vi "GetShortcuts.vi"(8 "error in (no error)":errorcluster, 11 "menu in":refnum<class "menu.lvclass">) -> (0 "error out":errorcluster, 2 "shortcuts":string[](array[string]), 3 "menu out":refnum<class "menu.lvclass">)   [LabVIEW 2009, in "menu.lvclass"]
uses:
  menu.lvclass
  menu.lvclass/menu.ctl
  Menu Item/menu item.lvclass
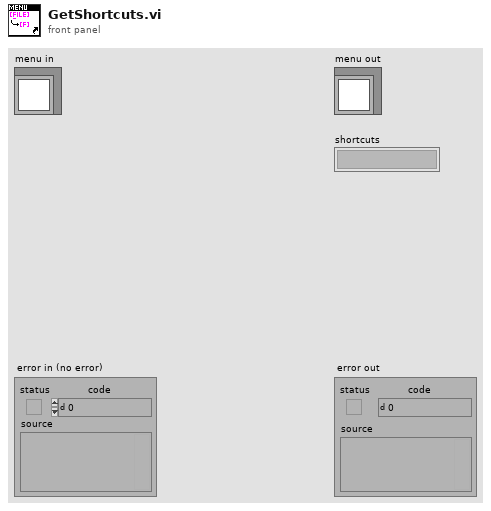
[diagram p1: front panel]
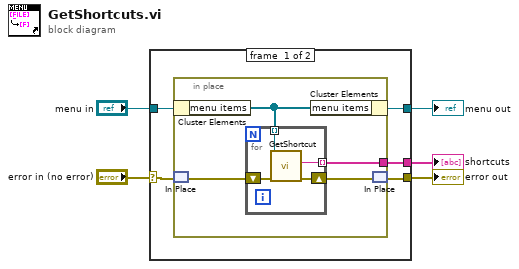
[diagram p0: block diagram]
diagram:
  n1 = case shown="No Error" "error in (no error)" {
    selector: "error in (no error)" -> [w7 w20]
    tunnel: [w8 w20] -> w2
    tunnel: [w9 w19] -> w4
    tunnel: "menu in" -> [w10 w19]
    tunnel: [w6 _] -> w1
    frame #0 {
      n2 = in-place {
        in-place-border: [w11] -> w6
        n3 = in-place-cluster #1(w10) -> ("menu items"=w14:refnum<class "menu item.lvclass">[])
        n4 = in-place-match #2(w7) -> (w13:errorcluster)
        n5 = for {
          shift-right: [w18] -> w12
          shift-left: w13 -> [w17]
          tunnel: w14 -> [w16] mode=indexing
          tunnel: [w15] -> w11 mode=indexing
          n6 = call-dynamic "GetShortcut.vi"("error in (no error)"=w17, "menu item in"=w16) -> ("error out"=w18:errorcluster, "shortcut"=w15:string)  [unwired: 7 in, 1 out]
        }
        n7 = in-place-cluster #1("menu items"=w14) -> (w9:refnum<class "menu.lvclass">)
        n8 = in-place-match #2(w12) -> (w8:errorcluster)
      }
    }
    frame #1 {
    }
  }
  "menu out" <- w4
  "error out" <- w2
  "shortcuts" <- w1
